vi "Initialize 6229.vi"(8 "error in (no error)":errorcluster) -> (0 "error out":errorcluster)   [LabVIEW 2015]
panel:
  in  "Placeholder":i32=4
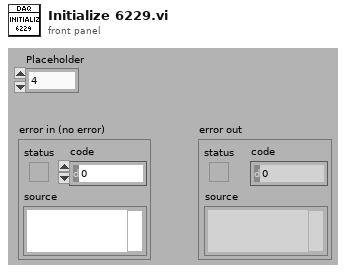
[diagram p1: front panel]
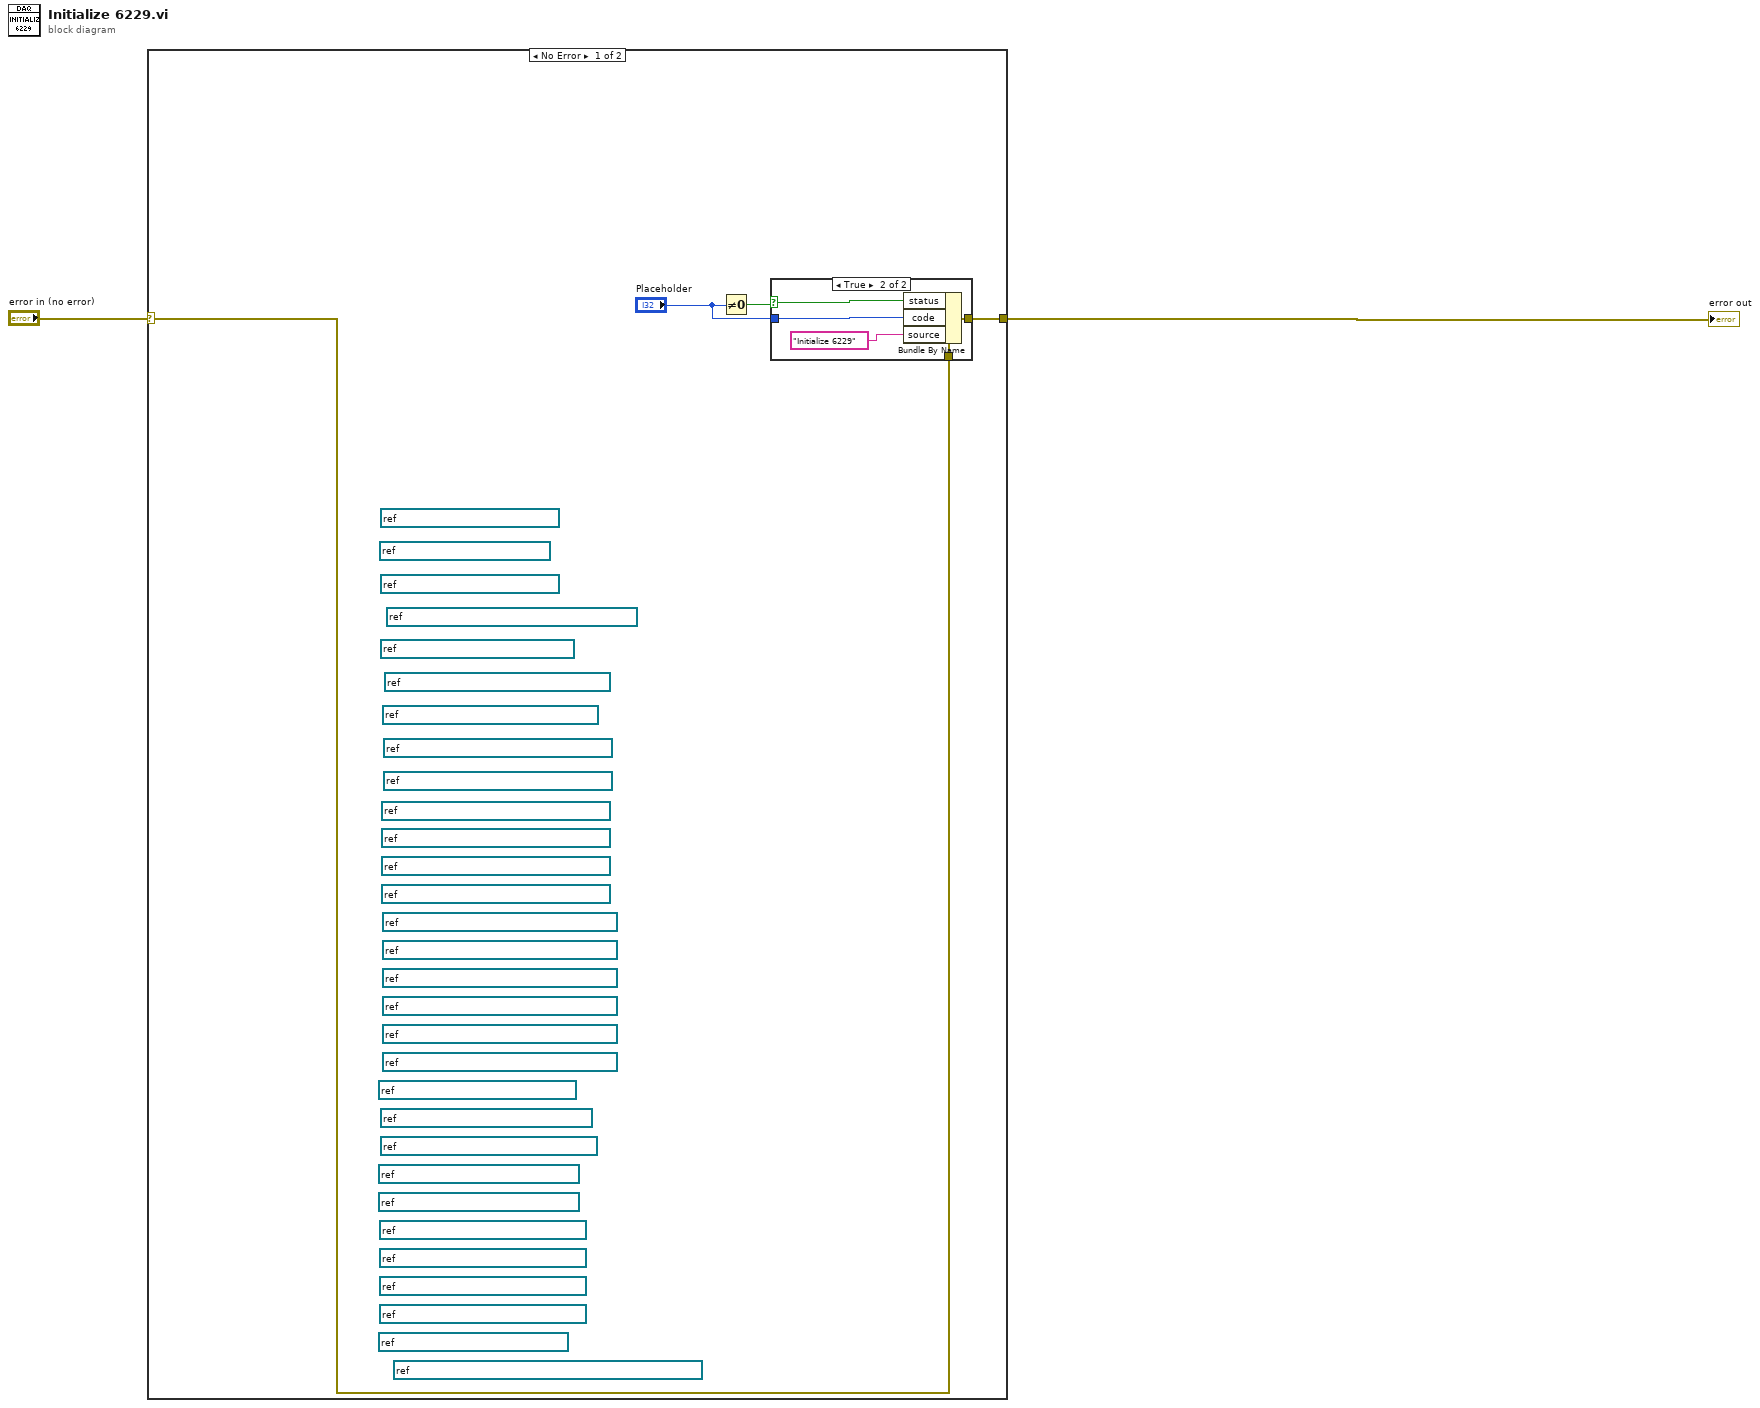
[diagram p0: block diagram]
diagram:
  n1 = case shown="No Error" "error in (no error)" {
    selector: "error in (no error)" -> [w5 w13]
    tunnel: [w6 w13] -> w1
    frame No Error {
      (unwired) refnum<k21> "MOC connect LIMITED2 to COMMON"
      (unwired) refnum<k21> "MOC connect LIMITED1 to COMMON"
      (unwired) refnum<k21> "MOC connect 440mA to COMMON"
      (unwired) refnum<k21> "ADC connect SW_BATT to COMMON"
      (unwired) refnum<k21> "ADC connect PS2 to COMMON"
      (unwired) refnum<k21> "ADC connect Power_Out_5V to COMMON"
      (unwired) refnum<k21> "ADC connect ID1 to Buss Bar"
      (unwired) refnum<k21> "ADC Connect ID1 to 5V VIC"
      (unwired) refnum<k21> "ADC connect ID0 to Buss Bar"
      (unwired) refnum<k21> "PSC connect RESERVED_AND_BANANA to COMMON"
      (unwired) refnum<k21> "PSC connect PS1 to VBATTERY"
      (unwired) refnum<k21> "PSC connect CAR14 to COMMON"
      (unwired) refnum<k21> "PSC connect CAR13 to COMMON"
      (unwired) refnum<k21> "PSC connect CAR12 to COMMON"
      (unwired) refnum<k21> "PSC connect CAR11 to COMMON"
      (unwired) refnum<k21> "PSC connect CAR9 to COMMON"
      (unwired) refnum<k21> "PSC connect CAR6 to COMMON"
      (unwired) refnum<k21> "PSC connect 160Ohm to COMMON"
      (unwired) refnum<k21> "OV connect 330Ohm to COMMON"
      (unwired) refnum<k21> "MOC connect PS1 to COMMON"
      (unwired) refnum<k21> "MOC connect LIMITED15 to COMMON"
      (unwired) refnum<k21> "MOC connect LIMITED14 to COMMON"
      (unwired) refnum<k21> "MOC connect LIMITED13 to COMMON"
      (unwired) refnum<k21> "MOC connect LIMITED12 to COMMON"
      (unwired) refnum<k21> "MOC connect LIMITED11 to COMMON"
      (unwired) refnum<k21> "MOC connect LIMITED10 to COMMON"
      (unwired) refnum<k21> "MOC connect LIMITED9 to COMMON"
      (unwired) refnum<k21> "MOC connect LIMITED8 to COMMON"
      (unwired) refnum<k21> "MOC connect LIMITED7 to COMMON"
      (unwired) refnum<k21> "MOC connect LIMITED6 to COMMON"
      n2 = Not Equal To 0?(x="Placeholder") -> (x != 0?=w4:bool)
      n3 = case shown="True" w4 {
        selector: w4 -> [_ w9]
        tunnel: [w7 w11] -> w6
        tunnel: w5 -> [w7 w10]
        tunnel: "Placeholder" -> [_ w8]
        frame False {
        }
        frame True {
          n4 = Bundle By Name(cluster=w10, "status"=w9, "code"=w8, "source"="Initialize 6229") -> (w11:errorcluster)
        }
      }
    }
    frame Error {
    }
  }
  "error out" <- w1
